vi "Serialize.vi"(8 "error in (no error)":errorcluster, 11 "VIP Publish In":refnum<class "VIP Publish.lvclass">) -> (0 "error out":errorcluster, 2 "Text":string)   [LabVIEW 2014, in "VIP Publish.lvclass"]
uses:
  VIP Publish.lvclass
  VIP Publish - STYP.ctl
  VIP Publish.lvclass/VIP Publish.ctl
  Read VIP_Path.vi
  Read Repo_Name.vi
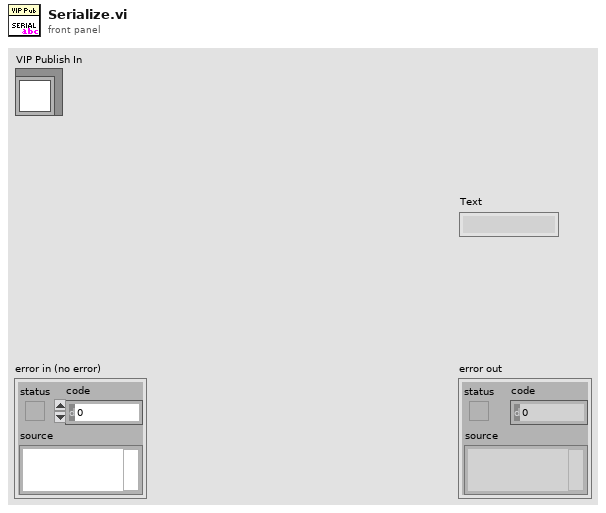
[diagram p1: front panel]
types:
  T1 = typedef "VIP Publish - STYP.ctl" = cluster{"VIP Path":string, "Repo Name":string}
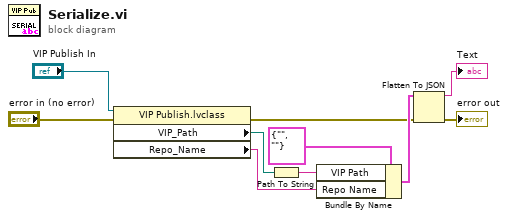
[diagram p0: block diagram]
diagram:
  n1 = property class="VIP Publish.lvclass"(reference="VIP Publish In", error in="error in (no error)") -> (error out=w5:errorcluster, "VIP_Path"=w8:path, "Repo_Name"=w1:string)  [unwired: 1 out]
  n2 = Path To String(path=w8) -> (string=w7:string)
  n3 = Bundle By Name(cluster=T1 {"VIP Path"="", "Repo Name"=""} ("VIP Publish"), "VIP Path"=w7, "Repo Name"=w1) -> (w6:T1)
  n4 = Flatten To JSON(anything=w6, error in (no error)=w5) -> (JSON string=→"Text":string, 11:→"error out":errorcluster)  [unwired: 1 in]
